vi "TestCountTimeouts.vi"() -> ()   [LabVIEW 2013]
panel:
  out "Waveform Graph":i16[][](graph)
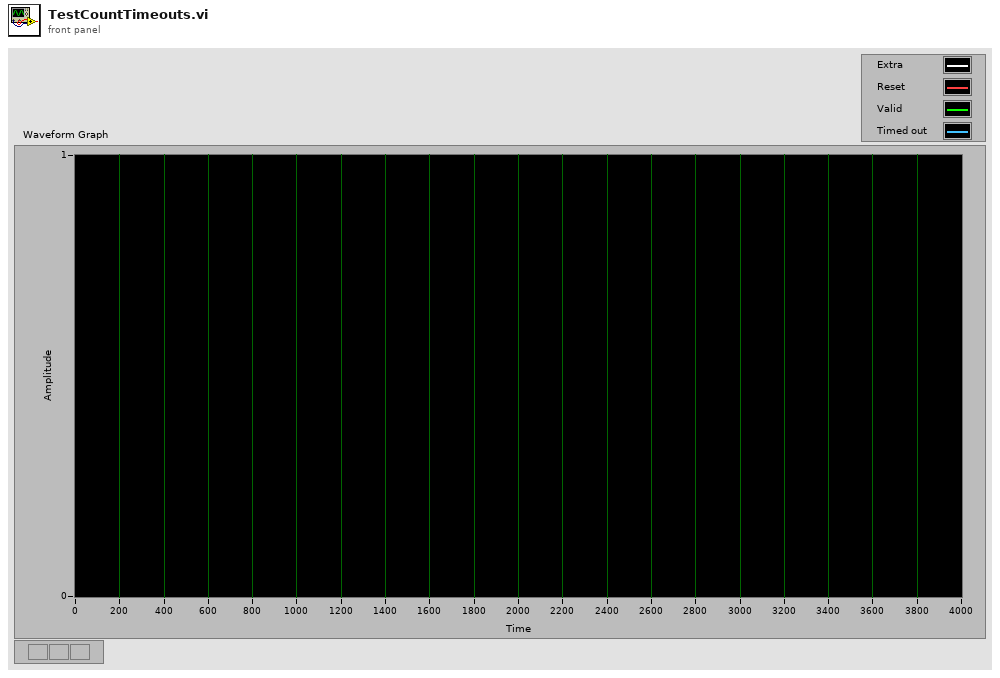
[diagram p1: front panel]
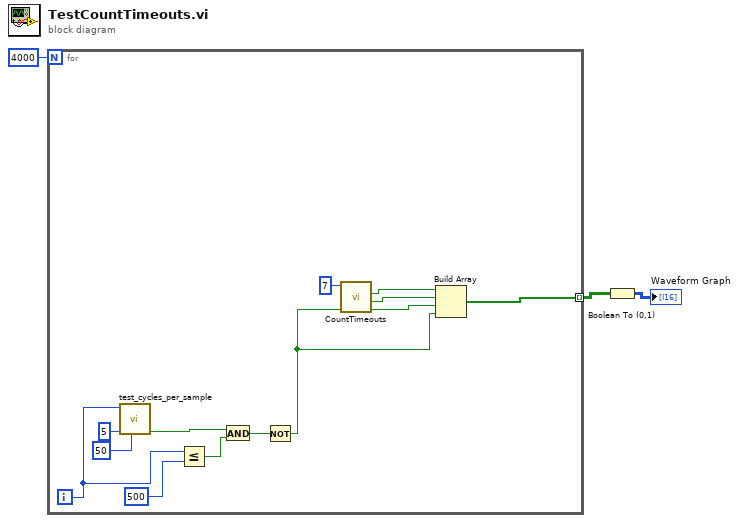
[diagram p0: block diagram]
diagram:
  n1 = for {
    N: 4000 -> [_]
    tunnel: [w6] -> w2 mode=indexing
    i -> [w13]
    n2 = call "test_cycles_per_sample.vi"("initial delay"=50, "cycles per sample"=5, "index"=w13) -> ("valid out"=w5:bool)  [unwired: 7 in, 1 out]
    n3 = Less Or Equal?(x=w13, y=500) -> (x <= y?=w11:bool)
    n4 = And(x=w5, y=w11) -> (x .and. y?=w10:bool)
    n5 = Not(x=w10) -> (.not. x?=w4:bool)
    n6 = call "CountTimeouts.vi"("Timed out"=w4, "Extra samples"=i16 7) -> ("Valid sample"=w7:bool, "Reset"=w8:bool, "Extra sample"=w9:bool)  [unwired: 7 in]
    n7 = Build Array(w9, w8, w7, w4) -> (w6:bool[])
  }
  n8 = Boolean To (0,1)(Boolean=w2) -> (0, 1=→"Waveform Graph":i16[][])
